vi "Get ctrl Secondary axis.vi"(3 "TypeDef":T1(array[ring])) -> (0 "Array":dbl[](array[numeric]))   [LabVIEW 2014]
uses:
  TypeDefs/SRE Enum.ctl
  Support Code/Robot Global Data.vi
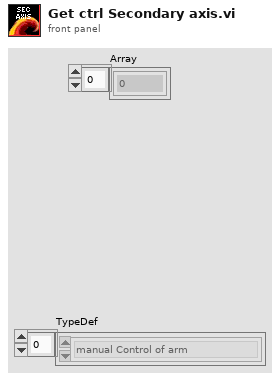
[diagram p1: front panel]
types:
  T1 = enum16{"manual Control of arm", "manual Control of Elevator", "Output Control"}[]
  T2 = typedef "SRE Enum.ctl" = enum16{"Start", "Run", "End"}
  T3 = enum16{"Left X", "Left Y", "Left trigger", "R trigger", "R X", "R Y"}[]
  T4 = enum16{"Left X", "Left Y", "Left trigger", "R trigger", "R X", "R Y"}
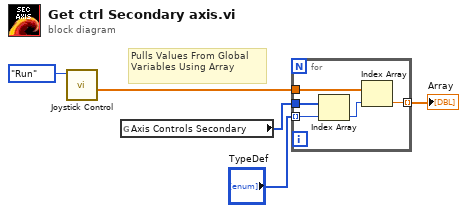
[diagram p0: block diagram]
diagram:
  # "Pulls Values From Global Variables Using Array"
  n1 = call "Joystick Control.vi"("Enum"=SRE_Enum."Run") -> ("Axis Output secondary"=w4:dbl[])  [unwired: 3 in, 5 out]
  n2 = global read "Robot Global Data.vi" "Axis Controls Secondary"() -> (w3:T3)
  n3 = for {
    tunnel: "TypeDef" -> [w10] mode=indexing
    tunnel: [w9] -> w2 mode=indexing
    tunnel: w4 -> [w8]
    tunnel: w3 -> [w6]
    n4 = Index Array(array=w6, index=w10) -> (element=w7:T4)
    n5 = Index Array(array=w8, index=w7) -> (element=w9:dbl)
  }
  "Array" <- w2
